vi "Compound_Boolean.vi"() -> ()   [LabVIEW 2019]
panel:
  out "result 2":bool
  out "result":bool
  in  "Boolean 10":bool
  in  "Boolean 9":bool
  in  "Boolean 7":bool
  in  "Boolean 6":bool
  in  "Boolean 5":bool
  in  "Boolean 3":bool
  in  "Boolean 2":bool
  in  "Boolean":bool
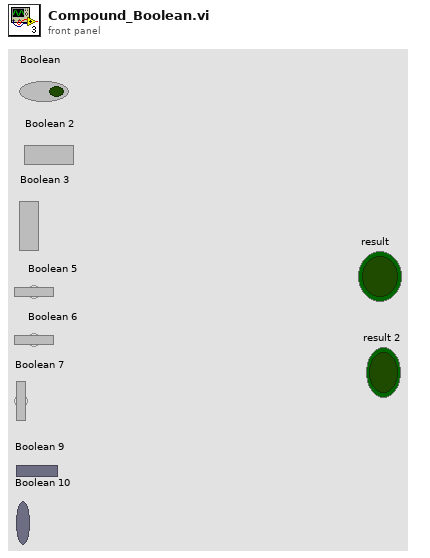
[diagram p1: front panel]
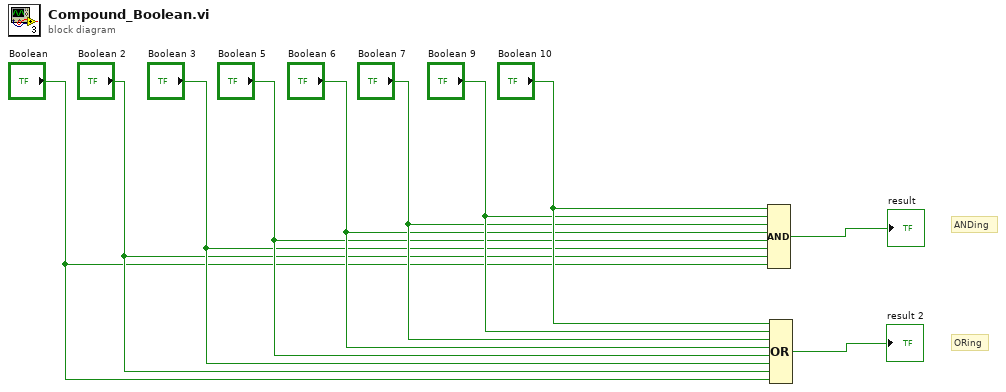
[diagram p0: block diagram]
diagram:
  # "ORing"
  # "ANDing"
  n1 = Compound Arithmetic op=AND("Boolean 10", "Boolean 9", "Boolean 7", "Boolean 6", "Boolean 5", "Boolean 3", "Boolean 2", "Boolean") -> (→"result":bool)
  n2 = Compound Arithmetic op=OR("Boolean 10", "Boolean 9", "Boolean 7", "Boolean 6", "Boolean 5", "Boolean 3", "Boolean 2", "Boolean") -> (→"result 2":bool)
